vi "XML_EEG_closeFile.vi"(8 "error in (no error)":errorcluster, 11 "XML_EEG_File.lvclass":refnum<class "XML_EEG_File.lvclass">) -> (0 "error out":errorcluster)   [LabVIEW 2016, in "XML_EEG_File_Parser.lvlib" / "XML_EEG_File.lvclass"]
uses:
  XML_EEG_File.lvclass
  XML_EEG_File.lvclass/XML_EEG_File.ctl
  <vilib>/xml/Close Reference(Node).vi
  <vilib>/xml/NI_XML.lvlib
panel:
  # "This VI is a part of BCI Design library, http://www.ru-bci.org \nCopyright © 2020, Sotnikov Peter, All rights reserved. License: CC BY-NC 4.0"
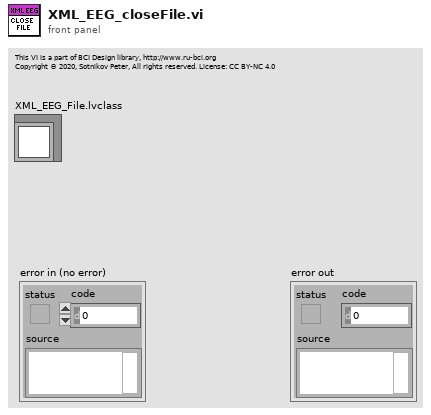
[diagram p1: front panel]
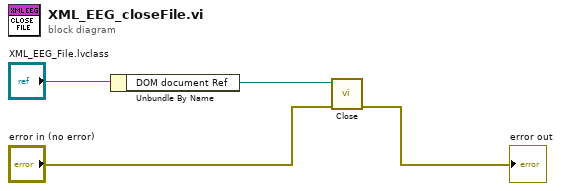
[diagram p0: block diagram]
diagram:
  n1 = Unbundle By Name("XML_EEG_File.lvclass") -> ("DOM document Ref"=w3:refnum<k20>)
  n2 = call-poly <vilib>:"Close.vi"("error in (no error)"="error in (no error)", "node"=w3) -> ("error out"=→"error out":errorcluster)  [unwired: 7 in]
